vi "pmu_Check PMU Location.vi"(8 "error in (no error)":errorcluster, 11 "CFG-3 PMU location":T1) -> (0 "error out":errorcluster, 3 "CFG-3 PMU location":T1)   [LabVIEW 2013, in "NI_EP_PMU.lvlib"]
uses:
  <vilib>/addons/Electrical Power/PMU/NI_EP_PMU.lvlib
  <vilib>/addons/Electrical Power/PMU/Common/Controls/pmu_CFG-3 PMU location.ctl
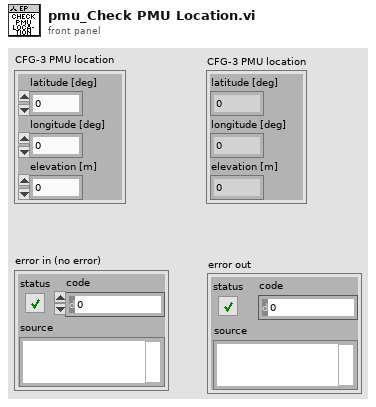
[diagram p1: front panel]
types:
  T1 = typedef "NI_EP_PMU.lvlib/pmu_CFG-3 PMU location.ctl" = cluster{"latitude [deg]":sgl, "longitude [deg]":sgl, "elevation [m]":sgl}
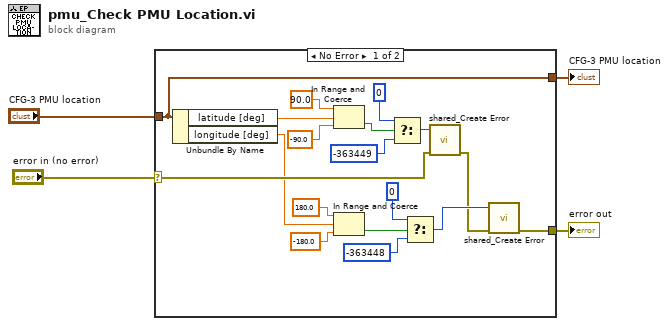
[diagram p0: block diagram]
diagram:
  n1 = case shown="No Error" "error in (no error)" {
    selector: "error in (no error)" -> [w18 _]
    tunnel: "CFG-3 PMU location" -> [w10 _]
    tunnel: [w11 _] -> w2
    tunnel: [w10 _] -> w1
    frame No Error {
      n2 = Unbundle By Name(w10) -> ("latitude [deg]"=w8:sgl, "longitude [deg]"=w17:sgl)
      n3 = In Range and Coerce(upper limit=sgl 90.0 ("latitude [deg]"), x=w8, lower limit=sgl -90.0 ("latitude [deg]")) -> (In Range?=w22:bool)  [unwired: 1 out]
      n4 = In Range and Coerce(upper limit=sgl 180.0 ("lower limit"), x=w17, lower limit=sgl -180.0) -> (In Range?=w14:bool)  [unwired: 1 out]
      n5 = Select(t=0, s=w22, f=-363449) -> (s? t:f=w19:i32)
      n6 = Select(t=0, s=w14, f=-363448) -> (s? t:f=w13:i32)
      n7 = call <vilib>:"shared_Create Error.vi"("error in (no error)"=w18, "error code (0)"=w19) -> ("error out"=w12:errorcluster)  [unwired: 9 in]
      n8 = call <vilib>:"shared_Create Error.vi"("error in (no error)"=w12, "error code (0)"=w13) -> ("error out"=w11:errorcluster)  [unwired: 9 in]
    }
    frame Error {
    }
  }
  "error out" <- w2
  "CFG-3 PMU location" <- w1
